vi "Ball HandlingPeriodic.vi"   [LabVIEW 2019]
uses:
  <vilib>/Rock Robotics/WPI/Solenoid/WPI_SolenoidValue.ctl
  <vilib>/Rock Robotics/WPI/Utilities/WPI_GetSetVariantRefNum.vi
  <vilib>/Rock Robotics/Network Tables/NT Read Boolean.vi
  <vilib>/Rock Robotics/WPI/Solenoid/WPI_SolenoidSetEnum.vi
  <vilib>/Rock Robotics/Network Tables/NT Write Boolean.vi
types:
  T1 = typedef "WPI_JoystickDevRef.ctl" = cluster{"Device":T2}
  T2 = typedef "WPI_JoystickDeviceEnum.ctl" = enum16{"USB 0", "USB 1", "USB 2", "USB 3", "USB 4", "USB 5"}
  T3 = typedef "WPI_SwitchDevRef.ctl" = cluster{"DevStatus":errorcluster, "DIO Channel":T4, "CntIndex":T5, "Normally Closed":bool}
  T4 = typedef "FPGA_DIOChannel.ctl" = enum8{"DIO 0", "DIO 1", "DIO 2", "DIO 3", "DIO 4", "DIO 5", "DIO 6", "DIO 7", "DIO 8", "DIO 9", "DIO MXP 0", "DIO MXP 1", "DIO MXP 2", "DIO MXP 3", "DIO MXP 4", "DIO MXP 5", "DIO MXP 6", "DIO MXP 7", "DIO MXP 8", "DIO MXP 9", "DIO MXP 10", "DIO MXP 11", "DIO MXP 12", "DIO MXP 13", "DIO MXP 14", "DIO MXP 15", "SPI Port CS1", "SPI Port CS2", "SPI Port CS3", "SPI Port MISO", "SPI Port MOSI", "Invalid"}
  T5 = typedef "FPGA_CounterCtrSystemIndex.ctl" = enum8{"Ctr 0", "Ctr 1", "Ctr 2", "Ctr 3", "Ctr 4", "Ctr 5", "Ctr 6", "Ctr 7", "Invalid"}
  T6 = typedef "WPI_MotorControlDeviceRef.ctl" = cluster{"DeviceStatus":errorcluster, "Type":T7, "PWM":cluster{"PWM Channel":T8, "DeadBand":T9}, "CAN":cluster{"Device Number":u8, "SetOutput VI Ref":variant, "GetOutput VI Ref":variant, "Enable VI Ref":variant, "Disable VI Ref":variant, "Data":variant}, "Invert":bool, "DIO PWM":cluster{"PWM \"Enable\" Channel":T8, "DIOChannel":T4, "PWM Rate":dbl}}
  T7 = typedef "WPI_MotorControlType.ctl" = enum16{"PWM", "CAN", "DIO PWM"}
  T8 = typedef "FPGA_DIOPWMChannel.ctl" = enum8{"PWM 0", "PWM 1", "PWM 2", "PWM 3", "PWM 4", "PWM 5", "PWM 6", "PWM 7", "PWM 8", "PWM 9", "PWM MXP 0", "PWM MXP 1", "PWM MXP 2", "PWM MXP 3", "PWM MXP 4", "PWM MXP 5", "PWM MXP 6", "PWM MXP 7", "PWM MXP 8", "PWM MXP 9", "Invalid"}
  T9 = typedef "WPI_PWMDeadband.ctl" = cluster{"Name":string, "maxPositivePwm":i32, "minPositivePwm":i32, "centerPwm":i32, "maxNegativePwm":i32, "minNegativePwm":i32, "angularRange":u16}
  T10 = typedef "WPI_SolenoidValue.ctl" = enum16{"Off", "On", "Forward", "Reverse"}
  T11 = typedef "WPI_SolenoidDevRef.ctl" = cluster{"DevStatus":errorcluster, "Pneumatics Control Module":u8, "Forward Solenoid Channel":T12, "Reverse Solenoid Channel":T12}
  T12 = typedef "WPI_SolenoidChannel.ctl" = enum8{"Solenoid 0", "Solenoid 1", "Solenoid 2", "Solenoid 3", "Solenoid 4", "Solenoid 5", "Solenoid 6", "Solenoid 7", "Invalid"}
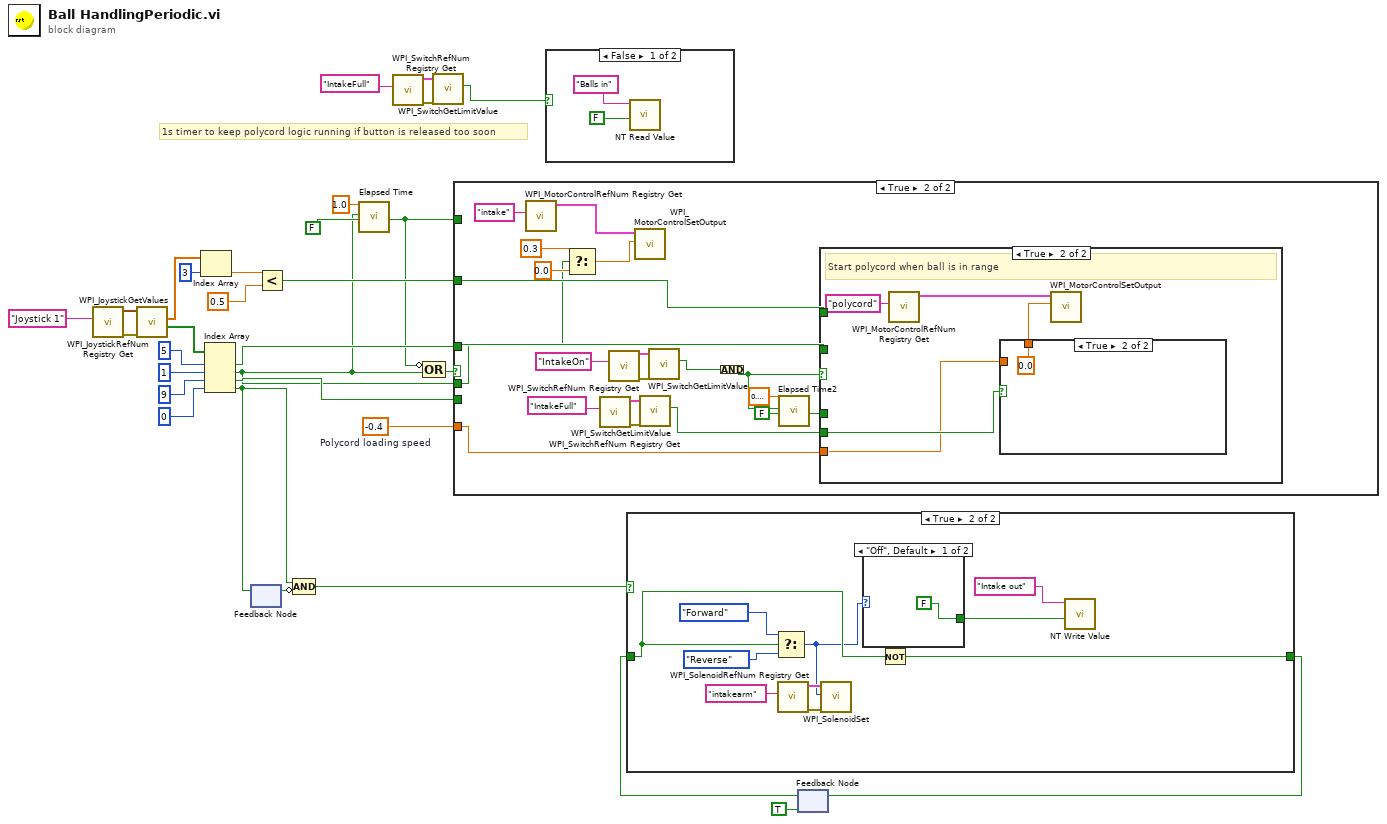
[diagram p0: block diagram]
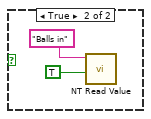
[diagram p2: hidden frame]
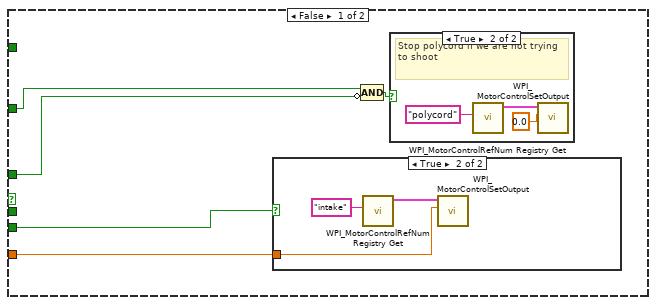
[diagram p3: hidden frame]
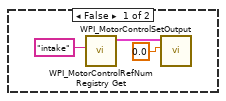
[diagram p5: hidden frame]
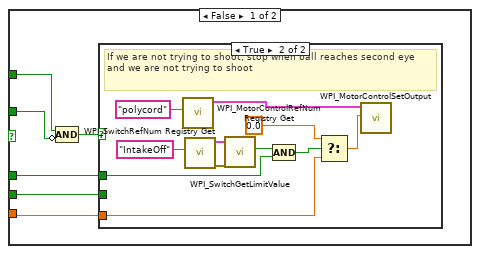
[diagram p6: hidden frame]
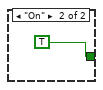
[diagram p10: hidden frame]
diagram:
  w5 = -0.4  # Polycord loading speed
  # "1s timer to keep polycord logic running if button is released too soon"
  n1 = call <vilib>:"WPI_JoystickRefNum Registry Get.vi"("refnum name"="Joystick 1") -> ("error out"=w30:errorcluster, "JoystickDevRef"=w29:T1)  [unwired: 9 in]
  n2 = call <vilib>:"WPI_JoystickGetValues.vi"("error in (no error)"=w30, "JoystickDevRef"=w29) -> ("Buttons"=w28:bool[], "Axes"=w15:dbl[])  [unwired: 5 in, 3 out]
  n3 = Index Array(array=w15, index=3) -> (element=w18:dbl)
  n4 = Index Array(array=w28, index #1=5 ("index"), index #2=1 ("index"), index #3=9 ("index"), index #4=0 ("index")) -> (element #1=w12:bool, element #2=w6:bool, element #3=w11:bool, element #4=w20:bool)
  n5 = feedback #1() -> (w19:bool)  [unwired: 1 in]
  n6 = feedback-in #1(w20) -> ()
  n7 = Less?(x=w18, y=0.5) -> (x < y?=w14:bool)
  n8 = Compound Arithmetic op=AND(w20, invert w19) -> (w22:bool)
  n9 = call "Elapsed Time"("Time Target (s)"=1.0, "Reset"=w6, "Auto Reset"=FALSE) -> ("Time has Elapsed"=w7:bool)  [unwired: 9 in, 7 out]
  n10 = call <vilib>:"WPI_SwitchRefNum Registry Get.vi"("refnum name"="IntakeFull") -> ("error out"=w3:errorcluster, "SwitchDevRef"=w4:T3)  [unwired: 9 in]
  n11 = Compound Arithmetic op=OR(invert w7, w6) -> (w8:bool)
  n12 = call <vilib>:"WPI_SwitchGetLimitValue.vi"("error in (no error)"=w3, "SwitchDevRef"=w4) -> ("Switch Pressed"=w1:bool)  [unwired: 7 in, 2 out]
  n13 = case shown="True" w8 {
    tunnel: w14 -> [w35 w61]
    tunnel: w12 -> [w34 w60]
    tunnel: w11 -> [w36 _]
    tunnel: w7 -> [_ _]
    tunnel: w6 -> [_ w52]
    tunnel: w5 -> [w32 w47]
    frame False {
      n14 = case shown="True" w36 {
        tunnel: w32 -> [_ w43]
        frame False {
          n15 = call <vilib>:"WPI_MotorControlRefNum Registry Get.vi"("refnum name"="intake") -> ("MotorControlDevRef"=w41:T6)  [unwired: 9 in, 1 out]
          n16 = call <vilib>:"WPI_MotorControlSetOutput.vi"("Output"=0.0, "MotorControlDevRef"=w41) -> ()  [unwired: 7 in, 3 out]
        }
        frame True {
          n17 = call <vilib>:"WPI_MotorControlRefNum Registry Get.vi"("refnum name"="intake") -> ("MotorControlDevRef"=w44:T6)  [unwired: 9 in, 1 out]
          n18 = call <vilib>:"WPI_MotorControlSetOutput.vi"("Output"=w43, "MotorControlDevRef"=w44) -> ()  [unwired: 7 in, 3 out]
        }
      }
      n19 = Compound Arithmetic op=AND(w35, invert w34) -> (w33:bool)
      n20 = case shown="True" w33 {
        frame False {
        }
        frame True {
          # "Stop polycord if we are not trying to shoot"
          n21 = call <vilib>:"WPI_MotorControlRefNum Registry Get.vi"("refnum name"="polycord") -> ("MotorControlDevRef"=w38:T6)  [unwired: 9 in, 1 out]
          n22 = call <vilib>:"WPI_MotorControlSetOutput.vi"("Output"=0.0, "MotorControlDevRef"=w38) -> ()  [unwired: 7 in, 3 out]
        }
      }
    }
    frame True {
      n23 = call <vilib>:"WPI_MotorControlRefNum Registry Get.vi"("refnum name"="intake") -> ("MotorControlDevRef"=w65:T6)  [unwired: 9 in, 1 out]
      n24 = Select(t=0.3 ("Output"), s=w52, f=0.0) -> (s? t:f=w54:dbl)
      n25 = call <vilib>:"WPI_SwitchRefNum Registry Get.vi"("refnum name"="IntakeFull") -> ("error out"=w63:errorcluster, "SwitchDevRef"=w64:T3)  [unwired: 9 in]
      n26 = call <vilib>:"WPI_SwitchRefNum Registry Get.vi"("refnum name"="IntakeOn") -> ("error out"=w59:errorcluster, "SwitchDevRef"=w58:T3)  [unwired: 9 in]
      n27 = call <vilib>:"WPI_MotorControlSetOutput.vi"("Output"=w54, "MotorControlDevRef"=w65) -> ()  [unwired: 7 in, 3 out]
      n28 = call <vilib>:"WPI_SwitchGetLimitValue.vi"("error in (no error)"=w63, "SwitchDevRef"=w64) -> ("Switch Pressed"=w46:bool)  [unwired: 7 in, 2 out]
      n29 = call <vilib>:"WPI_SwitchGetLimitValue.vi"("error in (no error)"=w59, "SwitchDevRef"=w58) -> ("Switch Pressed"=w56:bool)  [unwired: 7 in, 2 out]
      n30 = Compound Arithmetic op=AND(w56) -> (w51:bool)
      n31 = call "Elapsed Time2"("Time Target (s)"=0.20000000000000004, "Reset"=w51, "Auto Reset"=FALSE) -> ("Time has Elapsed"=w48:bool)  [unwired: 9 in, 7 out]
      n32 = case shown="True" w51 {
        tunnel: w61 -> [w71 _]
        tunnel: w60 -> [w70 _]
        tunnel: w47 -> [w69 w85]
        tunnel: w48 -> [w67 _]
        tunnel: w46 -> [w68 w86]
        frame False {
          n33 = Compound Arithmetic op=AND(w71, invert w70) -> (w72:bool)
          n34 = case shown="True" w72 {
            tunnel: w69 -> [_ w75]
            tunnel: w68 -> [_ _]
            tunnel: w67 -> [_ w73]
            frame False {
            }
            frame True {
              # "If we are not trying to shoot, stop when ball reaches second eye\nand we are not trying to shoot"
              n35 = call <vilib>:"WPI_MotorControlRefNum Registry Get.vi"("refnum name"="polycord") -> ("MotorControlDevRef"=w82:T6)  [unwired: 9 in, 1 out]
              n36 = call <vilib>:"WPI_SwitchRefNum Registry Get.vi"("refnum name"="IntakeOff") -> ("error out"=w80:errorcluster, "SwitchDevRef"=w81:T3)  [unwired: 9 in]
              n37 = call <vilib>:"WPI_SwitchGetLimitValue.vi"("error in (no error)"=w80, "SwitchDevRef"=w81) -> ("Switch Pressed"=w78:bool)  [unwired: 7 in, 2 out]
              n38 = Compound Arithmetic op=AND(w78, w73) -> (w74:bool)
              n39 = Select(t=0.0 ("Output"), s=w74, f=w75) -> (s? t:f=w76:dbl)
              n40 = call <vilib>:"WPI_MotorControlSetOutput.vi"("Output"=w76, "MotorControlDevRef"=w82) -> ()  [unwired: 7 in, 3 out]
            }
          }
        }
        frame True {
          # "Start polycord when ball is in range"
          n41 = call <vilib>:"WPI_MotorControlRefNum Registry Get.vi"("refnum name"="polycord") -> ("MotorControlDevRef"=w87:T6)  [unwired: 9 in, 1 out]
          n42 = case shown="True" w86 {
            tunnel: [w89 0.0 ("Polycord loading speed")] -> w84
            tunnel: w85 -> [w89 _]
            frame False {
            }
            frame True {
            }
          }
          n43 = call <vilib>:"WPI_MotorControlSetOutput.vi"("Output"=w84, "MotorControlDevRef"=w87) -> ()  [unwired: 7 in, 3 out]
        }
      }
    }
  }
  n44 = case shown="False" w1 {
    frame False {
      n45 = call-poly <vilib>:"NT Read Value.vi"("Default Value"=FALSE, "Name"="Balls in") -> ()  [unwired: 8 in, 2 out]
    }
    frame True {
      n46 = call-poly <vilib>:"NT Read Value.vi"("Default Value"=TRUE, "Name"="Balls in") -> ()  [unwired: 8 in, 2 out]
    }
  }
  n47 = feedback #2(TRUE) -> (w21:bool)
  n48 = case shown="True" w22 {
    tunnel: [w95 w100] -> w23
    tunnel: w21 -> [w95 w101]
    frame False {
    }
    frame True {
      n49 = Select(t=WPI_SolenoidValue."Forward" ("Value"), s=w101, f=WPI_SolenoidValue."Reverse") -> (s? t:f=w97:T10)
      n50 = call <vilib>:"WPI_SolenoidRefNum Registry Get.vi"("refnum name"="intakearm") -> ("error out"=w104:errorcluster, "SolenoidDevRef"=w103:T11)  [unwired: 9 in]
      n51 = call-poly <vilib>:"WPI_SolenoidSet.vi"("error in (no error)"=w104, "Value"=w97, "SolenoidDevRef"=w103) -> ()  [unwired: 7 in, 2 out]
      n52 = case shown="\"Off\", Default" w97 {
        tunnel: [FALSE ("Boolean") TRUE ("Boolean")] -> w96
        frame "Off", Default {
        }
        frame "On" {
        }
      }
      n53 = Not(x=w101) -> (.not. x?=w100:bool)
      n54 = call-poly <vilib>:"NT Write Value.vi"("Boolean"=w96, "Name"="Intake out") -> ()  [unwired: 9 in, 1 out]
    }
  }
  n55 = feedback-in #2(w23) -> ()
